vi "Read Holding Registers.vi"(6 "timeout ms (1000)":i32=1000, 8 "error in (no error)":errorcluster, 9 "Number of Registers":u16, 10 "Start Address":u16, 11 "Modbus TCP Micro Master in":refnum<class "Modbus TCP Micro Master.lvclass">) -> (0 "error out":errorcluster, 2 "Holding Registers":u16[](array[numeric]), 3 "Modbus TCP Micro Master out":refnum<class "Modbus TCP Micro Master.lvclass">)   [LabVIEW 2023, in "Modbus TCP Micro.lvlib" / "Modbus TCP Micro Master.lvclass"]
uses:
  Modbus TCP Micro Master.lvclass
  Modbus TCP Micro Master.lvclass/Modbus TCP Micro Master.ctl
  Raw/Read U16.vi
  Raw/Modbus Request.vi
  Modbus TCP Micro.lvlib
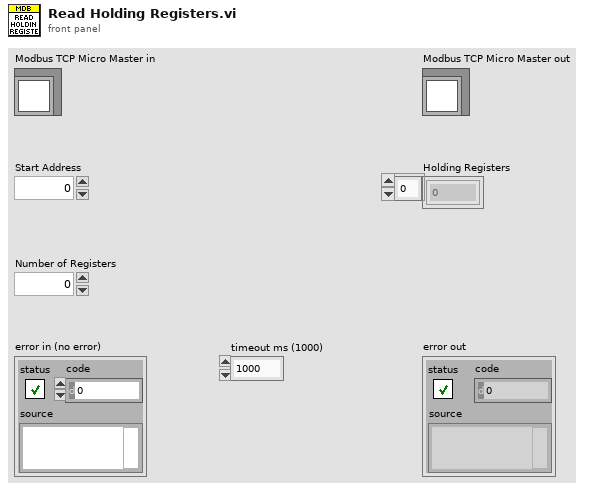
[diagram p1: front panel]
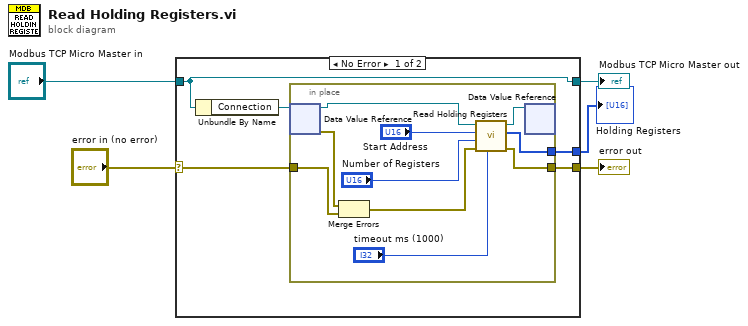
[diagram p0: block diagram]
diagram:
  n1 = case shown="No Error" "error in (no error)" {
    selector: "error in (no error)" -> [w8 w22]
    tunnel: [w7 w22] -> w4
    tunnel: [w10 w21] -> w2
    tunnel: "Modbus TCP Micro Master in" -> [w10 w21]
    tunnel: [w6 _] -> w1
    frame No Error {
      n2 = Unbundle By Name(w10) -> ("Connection"=w9:refnum<data-value>)
      n3 = in-place {
        in-place-border: w8 -> [w20]
        in-place-border: [w19] -> w7
        in-place-border: [w18] -> w6
        n4 = in-place-dvr #1(w9) -> (w17:refnum<k5>, w11:errorcluster)
        n5 = Merge Errors(w11, w20) -> (w12:errorcluster)
        n6 = call "Read Holding Registers.vi"("timeout ms (1000)"="timeout ms (1000)", "error in (no error)"=w12, "Number of Registers"="Number of Registers", "Start Address"="Start Address", "TCP Network Connection in"=w17) -> ("error out"=w19:errorcluster, "Array"=w18:u16[], "TCP Network Connection out"=w16:refnum<k5>)  [unwired: 4 in]
        n7 = in-place-dvr #1(w16) -> ()  [unwired: 2 out]
      }
    }
    frame Error {
    }
  }
  "error out" <- w4
  "Modbus TCP Micro Master out" <- w2
  "Holding Registers" <- w1
